vi "ReadPhysicsSettings.vi"   [LabVIEW 2020]
uses:
  <vilib>/Utility/config.llb/Read Key (Double).vi
  global/SettingVariable.vi
  <vilib>/Utility/config.llb/NI_LVConfig.lvlib
types:
  T1 = typedef "NI_LVConfig.lvlib/Config Data RefNum.ctl" = refnum<k1>
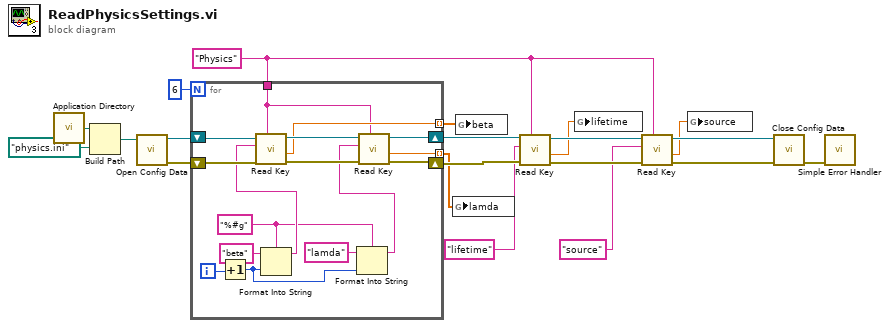
[diagram p0: block diagram]
diagram:
  w1 = "Physics"
  n1 = call <vilib>:"Application Directory.vi"() -> ("Application Directory"=w19:path)
  n2 = Build Path(base path=w19, name or relative path=path "physics.ini") -> (appended path=w18:path)
  n3 = call <vilib>:"Open Config Data.vi"("configuration file path"=w18) -> ("error out"=w15:errorcluster, "refnum"=w16:T1)  [unwired: 8 in, 1 out]
  n4 = for {
    N: 6 -> [_]
    tunnel: [w25] -> w12 mode=indexing
    tunnel: [w24] -> w11 mode=indexing
    shift-right: [w23] -> w13
    shift-left: w15 -> [w35]
    shift-right: [w22] -> w10
    shift-left: w16 -> [w36]
    tunnel: w1 -> [w21]
    i -> [w32]
    w27 = "%#g" ("format string")
    n5 = Increment(x=w32) -> (x+1=w29:i32)
    n6 = Format Into String(format string=w27, initial string="beta", w29) -> (resulting string=w30:string)  [unwired: 1 in, 1 out]
    n7 = call-poly <vilib>:"Read Key.vi"("section"=w21, "error in (no error)"=w35, "key"=w30, "refnum"=w36) -> ("error out"=w33:errorcluster, "value"=w25:dbl, "refnum out"=w34:T1)  [unwired: 4 in, 1 out]
    n8 = Format Into String(format string=w27, initial string="lamda", w29) -> (resulting string=w26:string)  [unwired: 1 in, 1 out]
    n9 = call-poly <vilib>:"Read Key.vi"("section"=w21, "error in (no error)"=w33, "key"=w26, "refnum"=w34) -> ("error out"=w23:errorcluster, "value"=w24:dbl, "refnum out"=w22:T1)  [unwired: 4 in, 1 out]
  }
  n10 = global write "SettingVariable.vi" "lamda"(w11) -> ()
  n11 = global write "SettingVariable.vi" "beta"(w12) -> ()
  n12 = call-poly <vilib>:"Read Key.vi"("section"=w1, "error in (no error)"=w13, "key"="lifetime" ("initial string"), "refnum"=w10) -> ("error out"=w7:errorcluster, "value"=w3:dbl, "refnum out"=w8:T1)  [unwired: 4 in, 1 out]
  n13 = global write "SettingVariable.vi" "lifetime"(w3) -> ()
  n14 = call-poly <vilib>:"Read Key.vi"("section"=w1, "error in (no error)"=w7, "key"="source" ("initial string"), "refnum"=w8) -> ("error out"=w5:errorcluster, "value"=w2:dbl, "refnum out"=w4:T1)  [unwired: 4 in, 1 out]
  n15 = global write "SettingVariable.vi" "source"(w2) -> ()
  n16 = call <vilib>:"Close Config Data.vi"("error in (no error)"=w5, "refnum"=w4) -> ("error out"=w14:errorcluster)  [unwired: 8 in, 1 out]
  n17 = call <vilib>:"Simple Error Handler.vi"("error in (no error)"=w14) -> ()  [unwired: 1 in, 8 out]
